vi "平台远程升级.vi"(8 "error in (no error)":errorcluster) -> (0 "error out":errorcluster)   [LabVIEW 2016, in "update.lvlib" / "http client.lvclass"]
uses:
  http client.lvclass
  update.lvlib
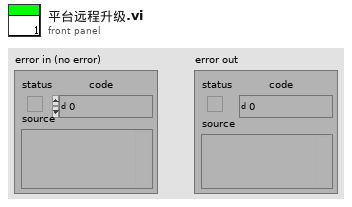
[diagram p1: front panel]
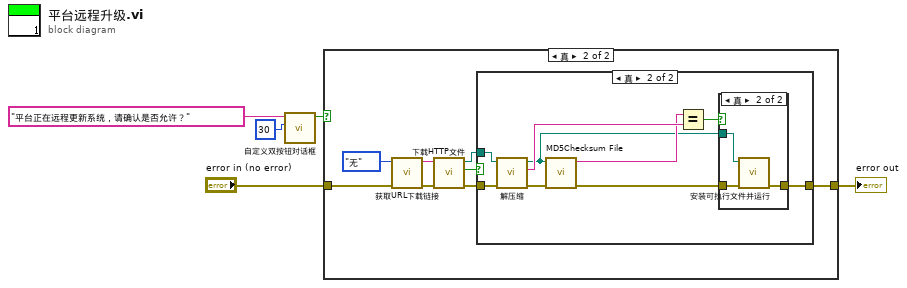
[diagram p0: block diagram]
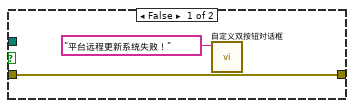
[diagram p3: hidden frame]
diagram:
  n1 = call "自定义双按钮对话框.vi"("数值"=30, "消息"="平台正在远程更新系统，请确认是否允许？") -> ("输出"=w3:bool)  [unwired: 9 in]
  n2 = case shown="真" w3 {
    tunnel: "error in (no error)" -> [w6 w9]
    tunnel: [w6 w8] -> w1
    frame False {
    }
    frame True {
      n3 = call "获取URL下载链接.vi"("error in (no error)"=w9, "固件升级"=enum16{"无", "CODMn", "氨氮", "总磷", "总氮", "CODCr"}."无") -> ("error out"=w12:errorcluster, "String/Binary data"=w11:string)  [unwired: 8 in]
      n4 = call "下载HTTP文件.vi"("error in (no error)"=w12, "Base URL"=w11) -> ("error out"=w13:errorcluster, "ok?"=w10:bool, "路径"=w14:path)  [unwired: 7 in]
      n5 = case shown="真" w10 {
        tunnel: w14 -> [_ w25]
        tunnel: w13 -> [w15 w24]
        tunnel: [w15 w17] -> w8
        frame False {
          n6 = call "自定义双按钮对话框.vi"("消息"="平台远程更新系统失败！") -> ()  [unwired: 10 in, 1 out]
        }
        frame True {
          n7 = call "解压缩.vi"("error in (no error)"=w24, "Zip file"=w25) -> ("error out"=w21:errorcluster, "MD5"=w23:string, "待校验的文件路径"=w20:path)  [unwired: 7 in]
          n8 = call <vilib>:"MD5Checksum File.vi"("error in (no error)"=w21, "Path"=w20) -> ("error out"=w19:errorcluster, "MD5 message-digest"=w22:string)  [unwired: 8 in]
          n9 = Equal?(x=w22, y=w23) -> (x = y?=w18:bool)
          n10 = case shown="真" w18 {
            tunnel: w20 -> [_ w29]
            tunnel: w19 -> [w26 w28]
            tunnel: [w26 w27] -> w17
            frame False {
            }
            frame True {
              n11 = call "安装可执行文件并运行.vi"("error in (no error)"=w28, "源路径"=w29) -> ("error out"=w27:errorcluster)  [unwired: 9 in]
            }
          }
        }
      }
    }
  }
  "error out" <- w1
